vi "Configure VIs for Development.vi"   [LabVIEW 2016, in "Static Error Handling.lvlib"]
uses:
  Static Error Handling.lvlib
types:
  T1 = enum32{"invalid VI type", "Standard VI", "Control VI", "Global VI", "Polymorphic VI", "Configuration VI", "SubSystem", "Facade VI", "Method VI", "Statechart Diagram VI"}
  T2 = enum16{"Share clones between instances", "Preallocate clone for each instance"}
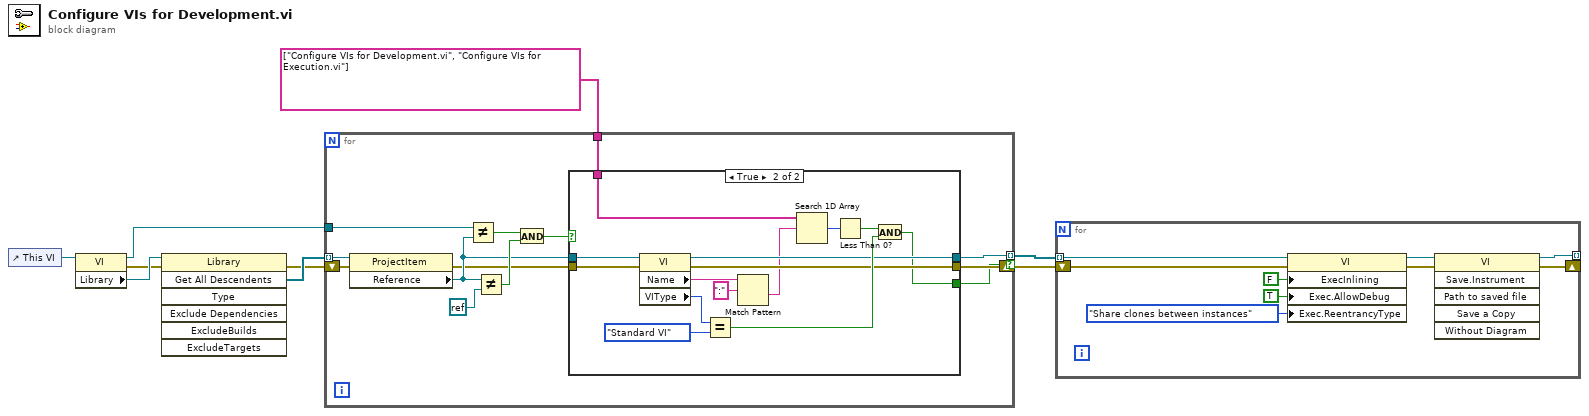
[diagram p0: block diagram]
diagram:
  n1 = control-ref of="This VI"() -> (w9:refnum<vi>)
  n2 = property class="VI"(reference=w9) -> (reference out=w8:refnum<vi>, error out=w1:errorcluster, "Library"=w5:refnum<vi>)  [unwired: 1 in]
  n3 = invoke class="Library" method="Get All Descendents"(reference=w5, error in=w1) -> (error out=w4:errorcluster, "All Descendents"=w6:refnum<vi>[])  [unwired: 5 in, 5 out]
  n4 = for {
    tunnel: w6 -> [w22] mode=indexing
    tunnel: [w14] -> w3 mode=indexing if=w12
    tunnel: w8 -> [w20]
    shift-right: [w13] -> w7
    shift-left: w4 -> [w18]
    tunnel: string[] ["Configure VIs for Development.vi", "Configure VIs for Execution.vi"] ("Blacklist VIs") -> [w10]
    n5 = property class="ProjectItem"(reference=w22, error in=w18) -> (error out=w15:errorcluster, "Reference"=w16:refnum<vi>)  [unwired: 1 out]
    n6 = Not Equal?(x=w20, y=w16) -> (x != y?=w19:bool)
    n7 = Not Equal?(x=w16, y=refnum<k0> refnum) -> (x != y?=w17:bool)
    n8 = And(x=w19, y=w17) -> (x .and. y?=w11:bool)
    n9 = case shown="True" w11 {
      selector: w11 -> [w24 _]
      tunnel: [w25 w30] -> w14
      tunnel: [w24 w27] -> w12
      tunnel: w16 -> [w25 w31]
      tunnel: [w23 w29] -> w13
      tunnel: w15 -> [w23 w32]
      tunnel: w10 -> [_ w28]
      frame False {
      }
      frame True {
        n10 = property class="VI"(reference=w31, error in=w32) -> (reference out=w30:refnum<vi>, error out=w29:errorcluster, "Name"=w33:string, "VIType"=w38:T1)
        n11 = Equal?(x=w38, y=T1."Standard VI" ("VI Type")) -> (x = y?=w35:bool)
        n12 = Match Pattern(string=w33, regular expression=":") -> (after substring=w26:string)  [unwired: 1 in, 3 out]
        n13 = Search 1D Array(1D array=w28, element=w26) -> (index of element=w37:i32)  [unwired: 1 in]
        n14 = Less Than 0?(x=w37) -> (x < 0?=w36:bool)
        n15 = And(x=w36, y=w35) -> (x .and. y?=w27:bool)
      }
    }
  }
  n16 = for {
    tunnel: w3 -> [w48] mode=indexing
    tunnel: [w41] -> _ mode=indexing
    shift-right: [w40] -> _
    shift-left: w7 -> [w47]
    n17 = property class="VI"(reference=w48, error in=w47, "ExecInlining"=FALSE ("Execution:Inline SubVI"), "Exec.AllowDebug"=TRUE ("Execution:Allow Debugging"), "Exec.ReentrancyType"=T2."Share clones between instances" ("Execution:Reentrancy Type")) -> (reference out=w42:refnum<vi>, error out=w43:errorcluster)
    n18 = invoke class="VI" method="Save.Instrument"(reference=w42, error in=w43) -> (reference out=w41:refnum<vi>, error out=w40:errorcluster)  [unwired: 4 in, 4 out]
  }
